vi "TLB Native Dynamic Events ver 0.05g.vi"() -> ()   [LabVIEW 2018]
uses:
  Labview Training Phase 2/Enum Controls/States for Action Engine.ctl
  Type def/TLB event states.ctl
  Type def/TLB MHL States.ctl
  <vilib>/Studica/Studica Toolkit/Background/I2C Channel.ctl
  <vilib>/Studica/Studica Toolkit/NavX/NavX.lvlib
  <vilib>/myRIO/Common/Instrument Driver Framework/myRIO v1.0/AI/typedefs/AI Channels Enum.ctl
  <vilib>/myRIO/Common/Instrument Driver Framework/myRIO v1.0/AI/typedefs/AI Channels List.ctl
  <vilib>/Studica/Studica Toolkit/Background/Mxp Selection.ctl
  <vilib>/ptbypt/NI_PtbyPt.lvlib
  Type def/Type def.ctl
  Type def/Motor Control Cluster.ctl
  <vilib>/Studica/Studica Blackhawk/Blackhawk.lvlib
  <vilib>/vision/driver/NI_Vision_Acquisition_Software.lvlib
  <vilib>/userdefined/High Color/IMAQdx.ctl
panel:
  in  "Enum":T1(ring)
  out "Image Processing error":errorcluster
  out "Image Out":T2(plugin-control)
  out "element":T3
  in  "Servo Angle":u8(slide) scale=0.0..180.0
  in  "On/Off":bool
  out "Blackhawk error":errorcluster
  out "Value Read":bool
  out "Object detected":bool
  out "Yaw":dbl
  in  "NavX Zero Yaw":bool
  out "NavX Info Out":T5
  out "LinearAcceleration":T6
  out "Displacement":T7
  out "YRPHfH":T8
  out "Distance":T9
  in  "Return to IDLE":bool
  out "Right IR Sensor":dbl
  out "Left IR Sensor":dbl
  out "CM":fxp<+,64,16>
  out "Ultrasonic sensor":dbl format="%0.2f"
  in  "xTargetSpeed":dbl
  in  "yTargetSpeed":dbl
  in  "wTargetSpeed":dbl
  out "Speed":T10
  in  "Reset Encoder 0":bool
  out "Action Queue Items":i32
  out "State Logic Queue Items":i32
  out "Action Queues items":string[](array[string])=["Hardware reset", "Software reset", ""]
  out "State logic":T11=enum."Task 2"
  out "Action State":string
  in  "Tasks Selector":string(combo)="Task 2"
  in  "Stop Queue":bool
  in  "Start Task":bool
  # "Test Programme written by Calvin Loke    Dated: 28 Aug 2019\nTest Programme revised by Dr Alex See   Dated 30 Aug 2019\n\nProgramme version:   TLB Native Dynamic Events ver 0.04b.vi"
  # "Sequence of Actions"
  # "Continuous (Repeated)"
  # "System Health Status Update"
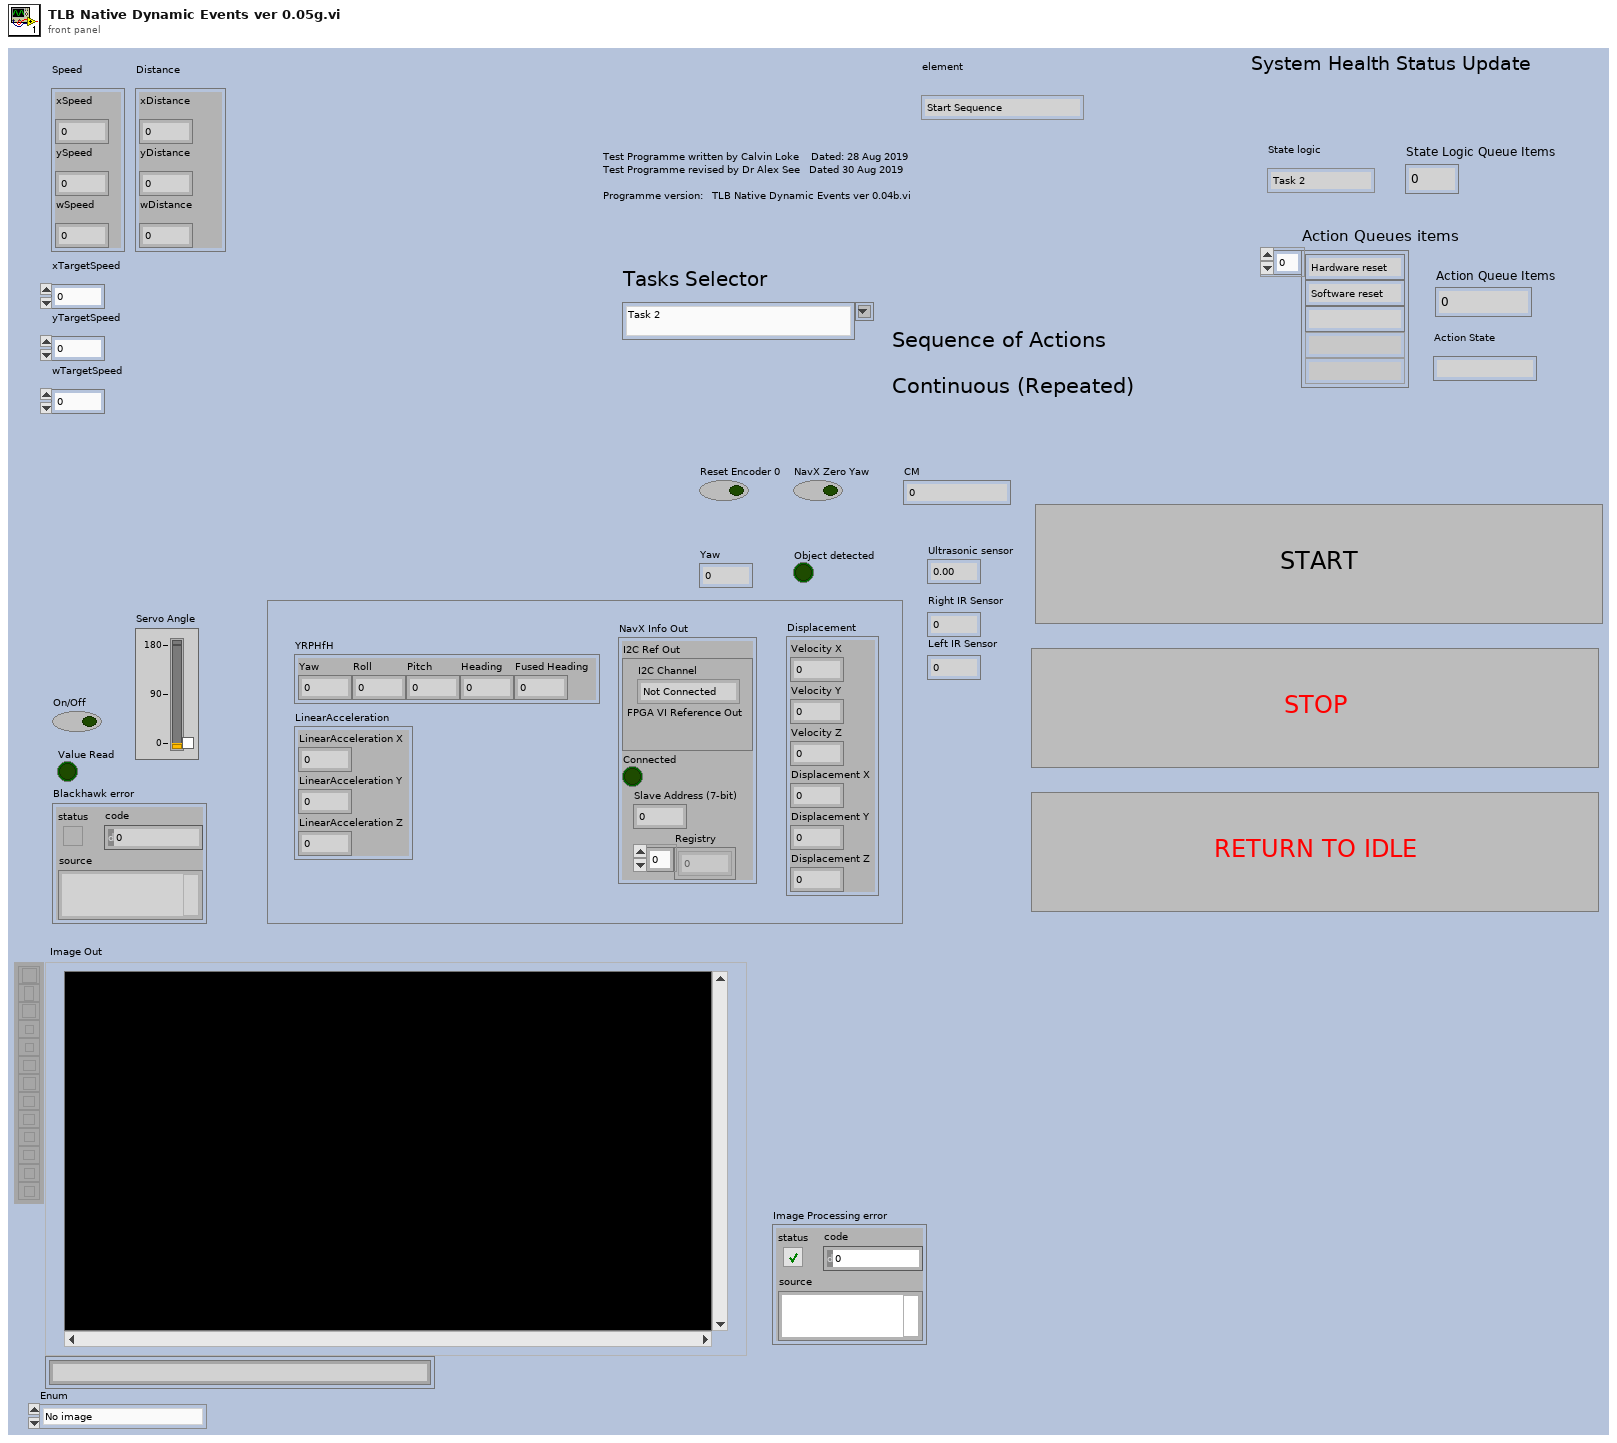
[diagram p1: front panel]
types:
  T1 = enum16{"No image", "Hair gel detection", "Pipe detection", "Ball detection", "Soap detection"}
  T2 = typedef "IMAQ Image.ctl" = refnum<image>
  T3 = typedef "TLB event states.ctl" = enum16{"Start Sequence", "Exit", "Start Task 1", "Start Task 2", "Start Task 3", "Start Task 4", "Camera vision", "Wall follow mode", "Idle", "Start Drive Straight"}
  T4 = typedef "I2C Channel.ctl" = enum16{"Not Connected", "A", "B"}
  T5 = cluster{"I2C Ref Out":cluster{"I2C Channel":T4, "FPGA VI Reference Out":refnum<k20>}, "Connected":bool, "Slave Address (7-bit)":u8, "Registry":u8[]}
  T6 = cluster{"LinearAcceleration X":dbl, "LinearAcceleration Y":dbl, "LinearAcceleration Z":dbl}
  T7 = cluster{"Velocity X":dbl, "Velocity Y":dbl, "Velocity Z":dbl, "Displacement X":dbl, "Displacement Y":dbl, "Displacement Z":dbl}
  T8 = cluster{"Yaw":dbl, "Roll":dbl, "Pitch":dbl, "Heading":dbl, "Fused Heading":dbl}
  T9 = cluster{"xDistance":dbl, "yDistance":dbl, "wDistance":dbl}
  T10 = cluster{"xSpeed":dbl, "ySpeed":dbl, "wSpeed":dbl}
  T11 = typedef "TLB MHL States.ctl" = enum16{"None", "Startup", "Idle", "Processing", "Shutdown", "Reset", "Task 1", "Task 2", "Task 3", "Task 4", "Task 4a", "Task 4b", "Task 4c", "Task 4d", "Task 4e", "Task 4f", "Task 4g", "Task 4h", "Acquire image", "Wall follow mode", "Autodrive", "Autodrive a"}
  T12 = typedef "States for Action Engine.ctl" = enum16{"Initialize", "Write", "Read"}
  T13 = typedef "IMAQdx.ctl" = refnum<k21>
  T14 = typedef "Motor Control Cluster.ctl" = cluster{"Vx":dbl, "Vy":dbl, "Vw":dbl}
  T15 = typedef "Type def.ctl" = cluster{"Front Ultrasonic Obstruct":bool, "Left Ultrasonic Obstruct":bool, "Right Ultrasonic Obstruct ":bool}
  T16 = typedef "Mxp Selection.ctl" = enum16{"MXP A", "MXP B"}
  T17 = typedef "TLB event states.ctl" = enum16{"Start Sequence", "Exit", "Start Task 1", "Start Task 2", "Start Task 3", "Start Task 4", "RT Camera tracking", "Wall follow mode", "Idle"}
  T18 = cluster{"I2C Channel":T4, "FPGA VI Reference Out":refnum<k20>}
  T19 = typedef "AI Channels List.ctl" = T20[]
  T20 = typedef "AI Channels Enum.ctl" = enum16{"Not Connected", "AudioIn/Left", "AudioIn/Right", "C/AI0", "C/AI1", "A/AI0", "A/AI1", "A/AI2", "A/AI3", "A/AI4", "A/AI5", "A/AI6", "A/AI7", "B/AI0", "B/AI1", "B/AI2", "B/AI3", "B/AI4", "B/AI5", "B/AI6", "B/AI7", "AI/AI0", "AI/AI1", "AI/AI2", "AI/AI3", "A/AI0 (DIFF)", "A/AI1 (DIFF)", "A/AI2 (DIFF)", "A/AI3 (DIFF)", "B/AI0 (DIFF)", "B/AI1 (DIFF)", "B/AI2 (DIFF)", "B/AI3 (DIFF)"}
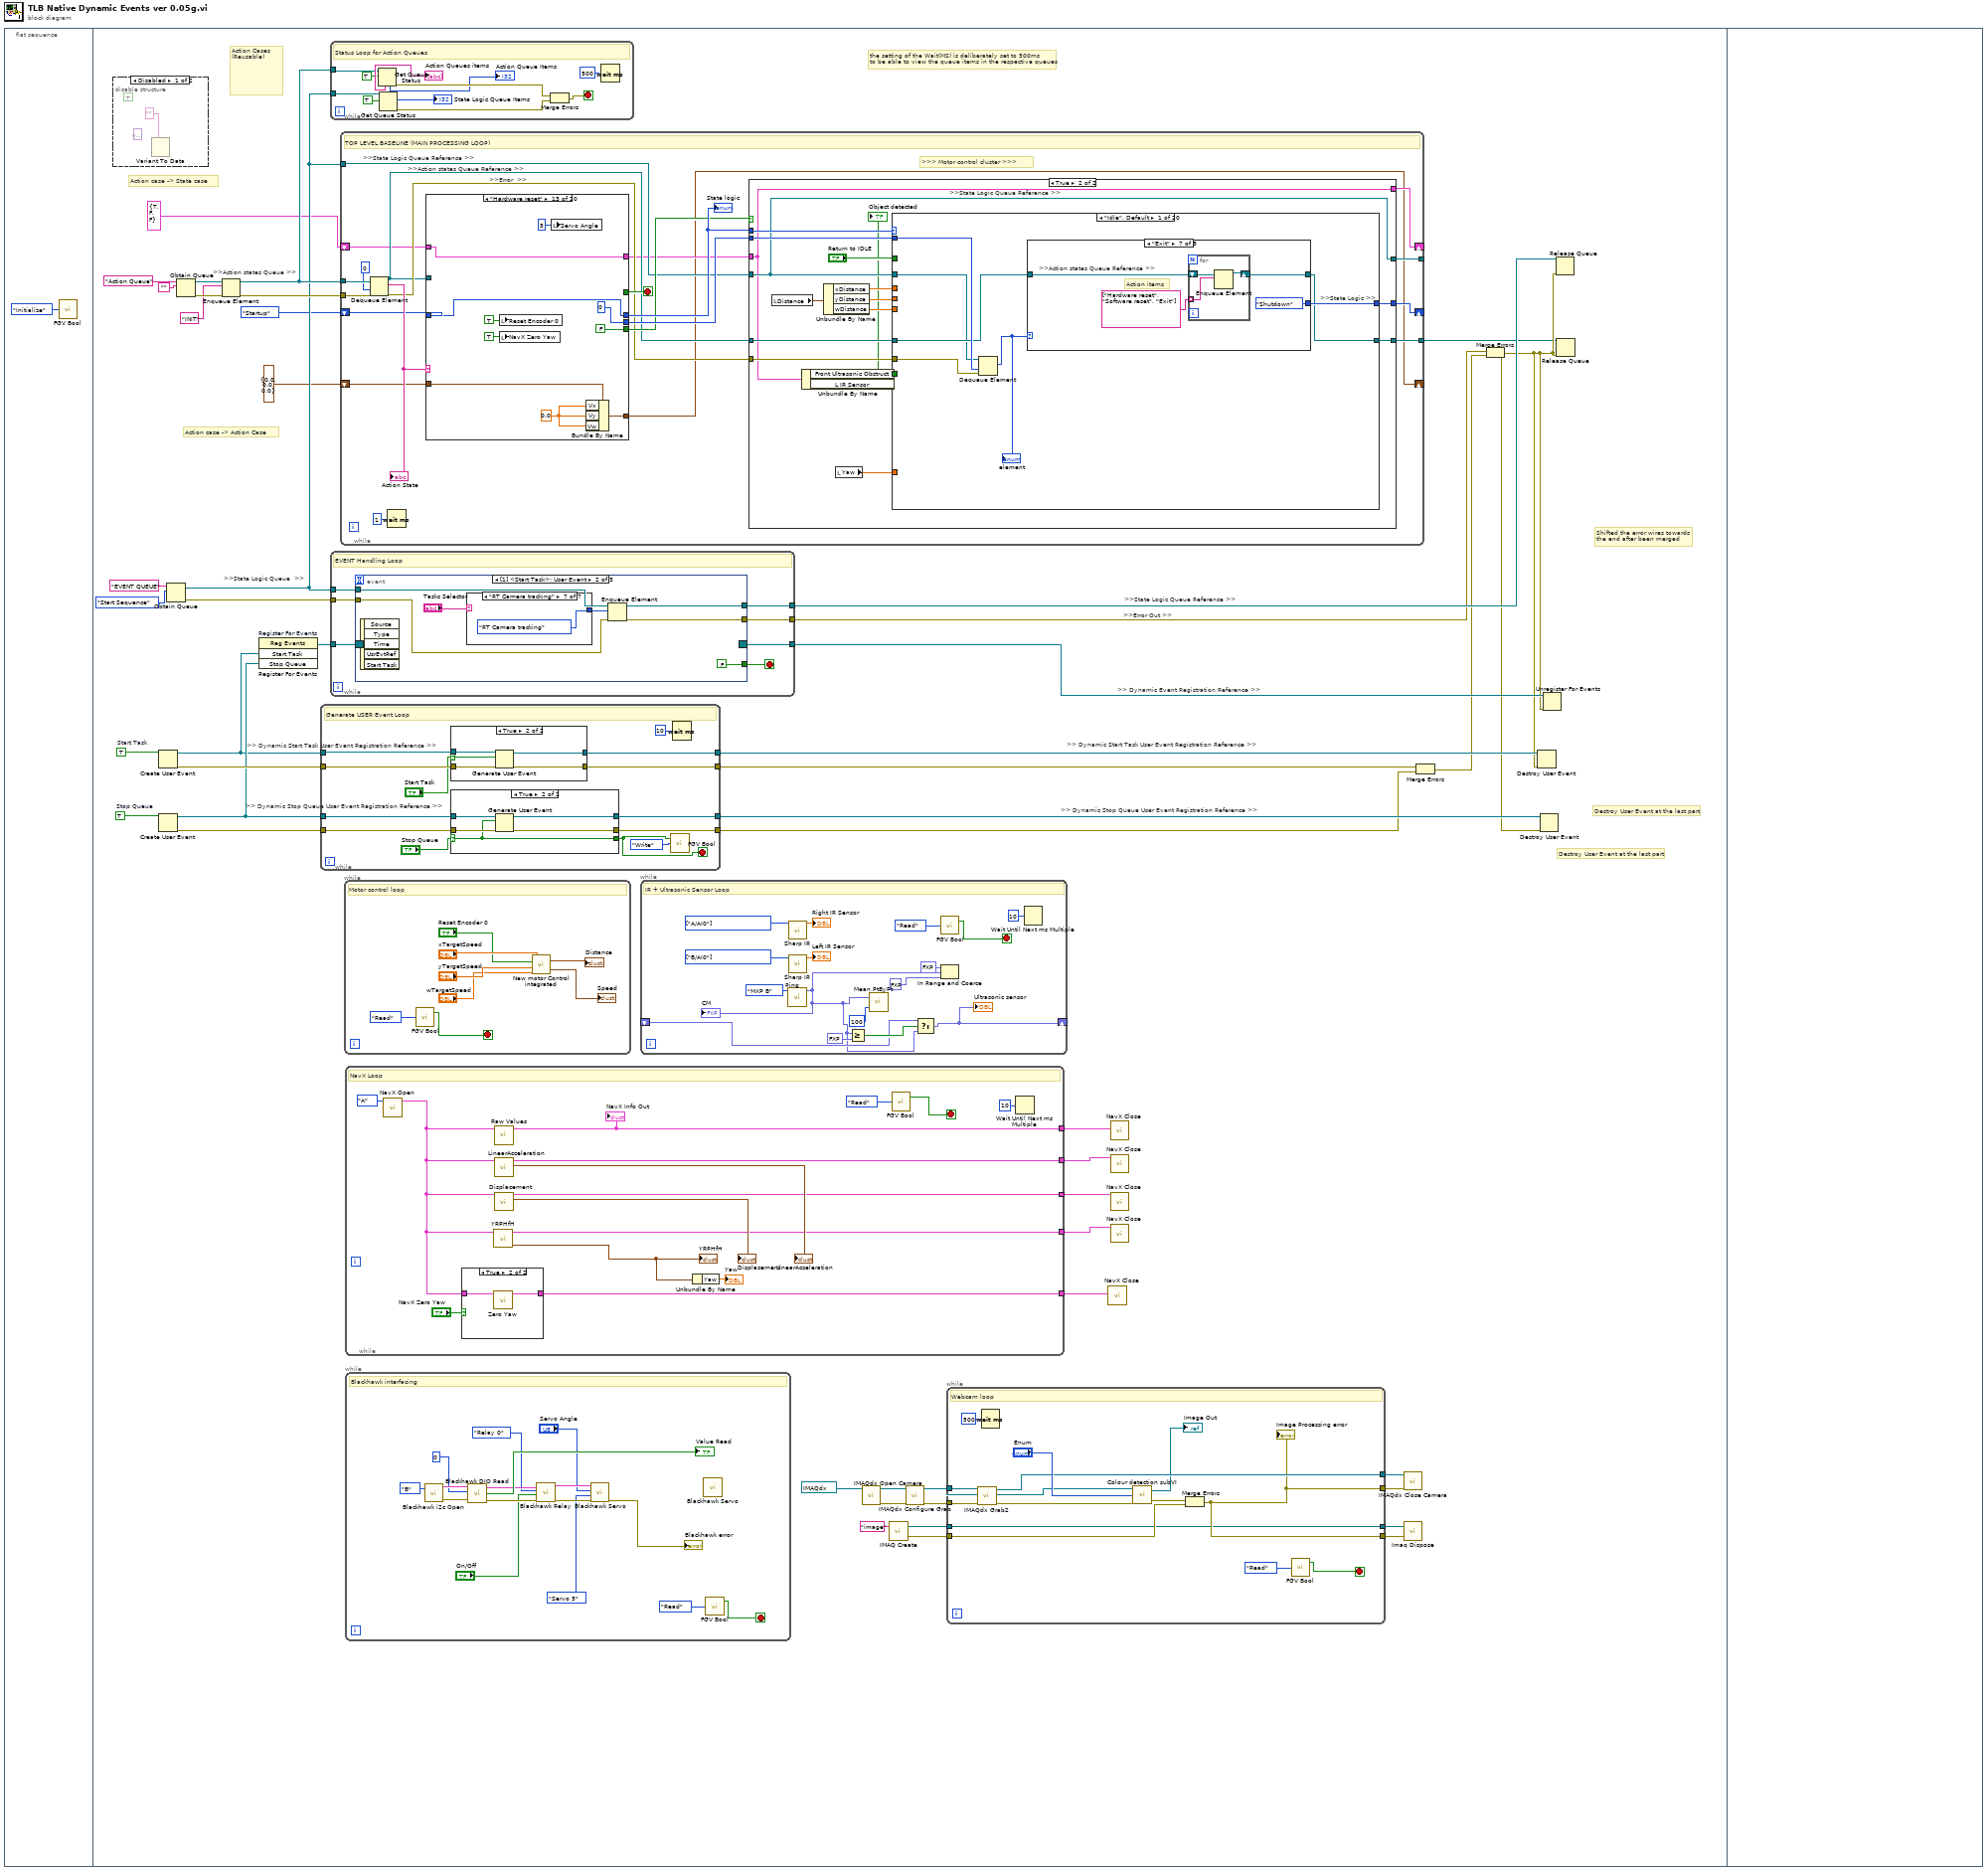
[diagram p0: block diagram]
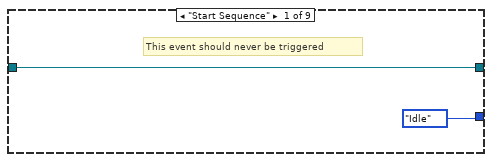
[diagram p5: hidden frame]
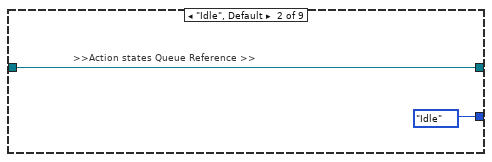
[diagram p6: hidden frame]
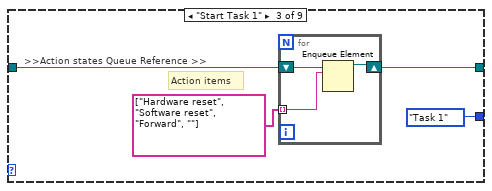
[diagram p7: hidden frame]
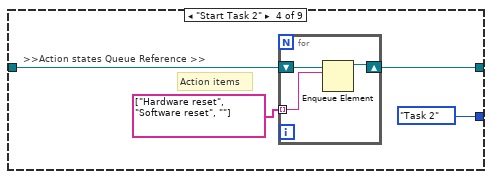
[diagram p8: hidden frame]
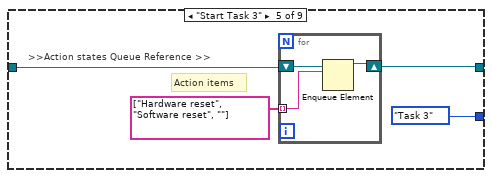
[diagram p9: hidden frame]
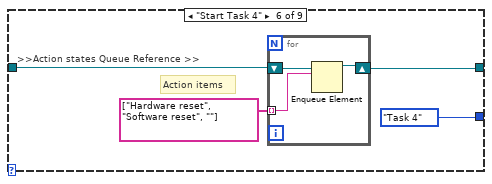
[diagram p10: hidden frame]
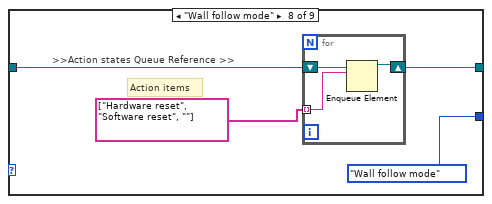
[diagram p11: hidden frame]
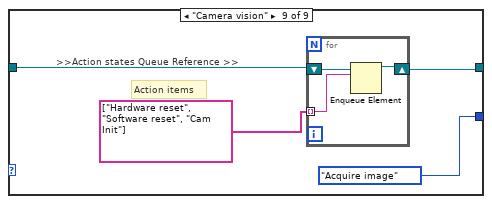
[diagram p12: hidden frame]
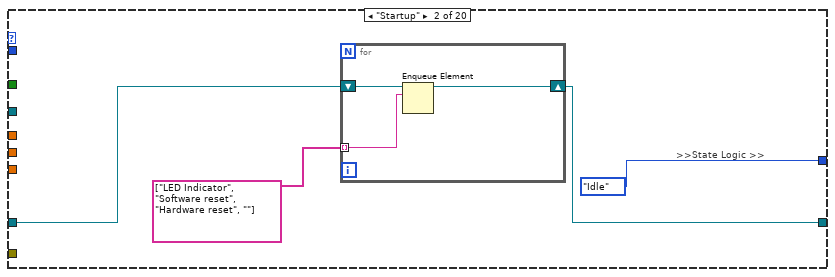
[diagram p13: hidden frame]
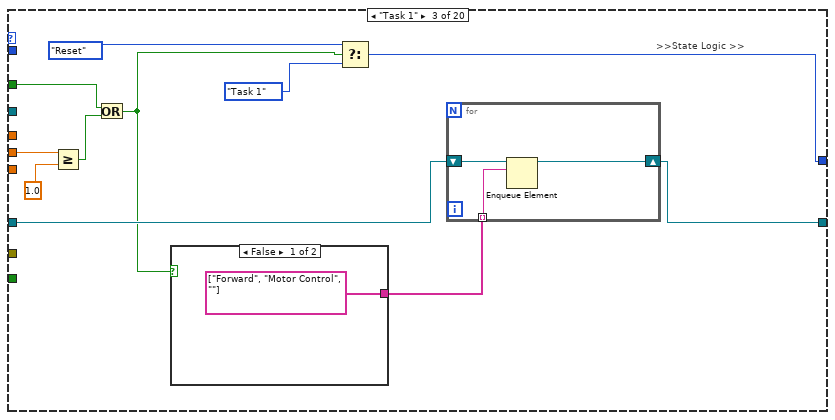
[diagram p14: hidden frame]
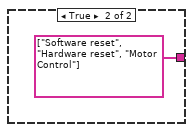
[diagram p15: hidden frame]
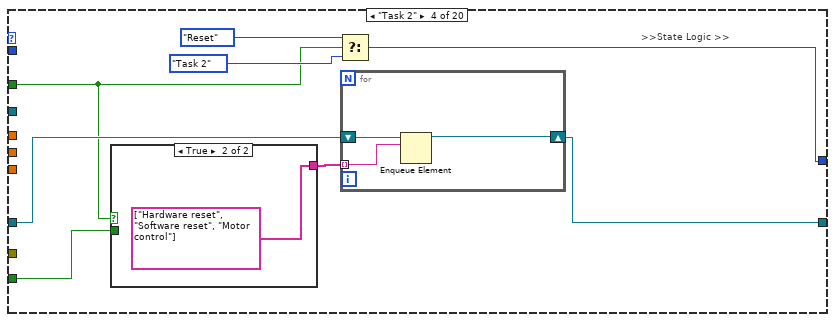
[diagram p16: hidden frame]
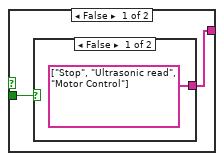
[diagram p17: hidden frame]
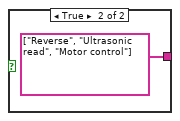
[diagram p18: hidden frame]
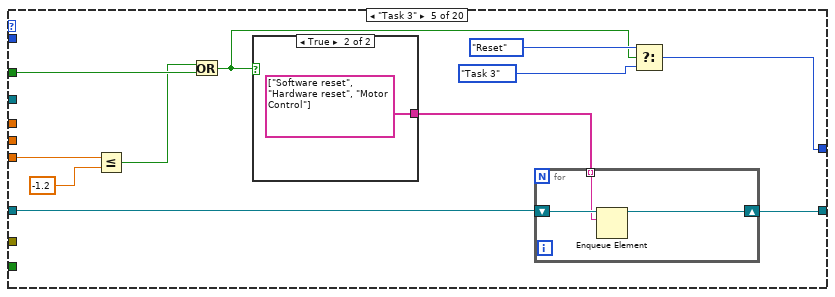
[diagram p19: hidden frame]
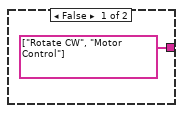
[diagram p20: hidden frame]
diagram:
  n1 = flat-sequence {
    frame #0 {
      n2 = call "FGV Bool.vi"("Init/Read/Write State"=States_for_Action_Engine."Initialize") -> ()  [unwired: 2 in, 2 out]
    }
    frame #1 {
      w49 = TRUE  # Stop Queue
      w48 = TRUE  # Start Task
      # "Action case -> Action Case"
      # "Action case -> State case"
      # "the setting of the Wait(MS) is deliberately set to 500ms\nto be able to view the queue items in the respective queues"
      # "Action Cases\n(Reusable)"
      # ">>Error Out >>"
      # ">> Dynamic Stop Queue User Event Registration Reference >>"
      # ">> Dynamic Start Task User Event Registration Reference >>"
      # ">> Dynamic Stop Queue User Event Registration Reference >>"
      # ">> Dynamic Start Task User Event Registration Reference >>"
      # ">> Dynamic Event Registration Reference >>"
      # ">>Action states Queue >>"
      # ">>State Logic Queue  >>"
      # ">>State Logic Queue Reference >>"
      # "Destroy User Event at the last part"
      # "Destroy User Event at the last part"
      # "Shifted the error wires towards\nthe end after been merged"
      n3 = disable-structure shown="Disabled" {
        frame Disabled {
          (unwired) variant
          (unwired) TRUE
          n4 = Variant To Data(type="") -> ()  [unwired: 2 in, 2 out]
        }
        frame Enabled {
        }
      }
      n5 = Create User Event(user event datatype=w48) -> (user event=w40:refnum<user-event>, error out=w45:errorcluster)  [unwired: 1 in]
      n6 = Create User Event(user event datatype=w49) -> (user event=w41:refnum<user-event>, error out=w44:errorcluster)  [unwired: 1 in]
      n7 = Obtain Queue(name (unnamed)="EVENT QUEUE", element data type=TLB_event_states."Start Sequence" ("Enum")) -> (queue out=w25:refnum<queue>, error out=w31:errorcluster)  [unwired: 3 in, 1 out]
      n8 = Obtain Queue(name (unnamed)="Action Queue", element data type="") -> (queue out=w34:refnum<queue>, error out=w30:errorcluster)  [unwired: 3 in, 1 out]
      n9 = Enqueue Element(queue=w34, element="INIT", error in (no error)=w30) -> (queue out=w26:refnum<queue>, error out=w29:errorcluster)  [unwired: 1 in, 1 out]
      n10 = register-events "Register For Events"(w40, w41) -> (reference out=w39:refnum<event-registration>)  [unwired: 2 in, 1 out]
      n11 = while {
        tunnel: w40 -> [w607]
        tunnel: w41 -> [w606]
        tunnel: [w605] -> w47
        tunnel: [w604] -> w46
        tunnel: w45 -> [w603]
        tunnel: [w602] -> w43
        tunnel: w44 -> [w601]
        tunnel: [w600] -> w42
        stop <- w596 stop-if-true
        # "Generate USER Event Loop"
        n12 = case shown="True" "Start Task" {
          selector: "Start Task" -> [_ w619]
          tunnel: w607 -> [w618 w623]
          tunnel: [w618 w622] -> w604
          tunnel: w603 -> [w617 w621]
          tunnel: [w617 w620] -> w602
          frame False {
          }
          frame True {
            n13 = Generate User Event(user event=w623, event data cluster=w619, error in=w621) -> (user event out=w622:refnum<user-event>, error out=w620:errorcluster)  [unwired: 1 in]
          }
        }
        n14 = case shown="True" "Stop Queue" {
          selector: "Stop Queue" -> [_ w612]
          tunnel: w606 -> [w611 w616]
          tunnel: [w611 w615] -> w605
          tunnel: w601 -> [w610 w614]
          tunnel: [w610 w613] -> w600
          tunnel: [FALSE w612] -> w596
          frame False {
          }
          frame True {
            n15 = Generate User Event(user event=w616, event data cluster=w612, error in=w614) -> (user event out=w615:refnum<user-event>, error out=w613:errorcluster)  [unwired: 1 in]
          }
        }
        n16 = call "FGV Bool.vi"("Init/Read/Write State"=States_for_Action_Engine."Write", "Input Node"=w596) -> ()  [unwired: 1 in, 2 out]
        n17 = Wait (ms)(milliseconds to wait=u32 10) -> ()  [unwired: 1 out]
      }
      n18 = while {
        tunnel: w26 -> [w131]
        tunnel: w25 -> [w128]
        stop <- w125 stop-if-true
        # "Status Loop for Action Queues"
        n19 = Get Queue Status(queue=w131, return elements? (F)=TRUE) -> (error out=w127:errorcluster, # elements in queue=→"Action Queue Items":i32, elements=→"Action Queues items":string[])  [unwired: 1 in, 5 out]
        n20 = Get Queue Status(queue=w128, return elements? (F)=TRUE) -> (# pending remove=→"State Logic Queue Items":i32, error out=w126:errorcluster)  [unwired: 1 in, 6 out]
        n21 = Merge Errors(w127, w126) -> (w125:errorcluster)
        n22 = Wait (ms)(milliseconds to wait=u32 500) -> ()  [unwired: 1 out]
      }
      n23 = while {
        tunnel: w39 -> [w569]
        tunnel: [w568] -> w38
        tunnel: w25 -> [w566]
        tunnel: [w565] -> w37
        tunnel: w31 -> [w564]
        tunnel: [w563] -> w28
        stop <- w567 stop-if-true
        # "EVENT Handling Loop"
        n24 = event shown="[1] <Start Task>: User Event" {
          selector: w569 -> [_ _ _]
          dyn-events: [_ _ _] -> w568
          timeout: _ -> [_ _ _]
          tunnel: [FALSE FALSE w595] -> w567
          tunnel: w566 -> [w574 w581 w593]
          tunnel: [w573 w580 w594] -> w565
          tunnel: w564 -> [w571 w577 w591]
          tunnel: [w570 w576 w590] -> w563
          event Timeout {
            n25 = event-data() -> ()  [unwired: 1 in, 3 out]
            n26 = Enqueue Element(queue=w574, element=TLB_event_states."Idle" ("Enum"), error in (no error)=w571) -> (queue out=w573:refnum<queue>, error out=w570:errorcluster)  [unwired: 1 in, 1 out]
          }
          event User Event {
            n27 = event-data() -> ()  [unwired: 1 in, 5 out]
            n28 = case shown="\"RT Camera tracking\"" "Tasks Selector" {
              tunnel: [TLB_event_states."Idle" ("Enum") TLB_event_states."Start Task 1" ("Enum") TLB_event_states."Start Task 2" ("Enum") TLB_event_states."Start Task 3" ("Enum") TLB_event_states."Start Task 4" ("Enum") TLB_event_states."Wall follow mode" ("Enum") TLB_event_states."RT Camera tracking" ("Enum")] -> w578
              frame Default {
              }
              frame "Task 1" {
              }
              frame "Task 2" {
              }
              frame "Task 3" {
              }
              frame "Task 4" {
              }
              frame "Wall following" {
              }
              frame "RT Camera tracking" {
              }
            }
            n29 = Enqueue Element(queue=w581, element=w578, error in (no error)=w577) -> (queue out=w580:refnum<queue>, error out=w576:errorcluster)  [unwired: 1 in, 1 out]
          }
          event User Event {
            n30 = event-data() -> ("Stop Queue"=w595:bool)  [unwired: 1 in, 4 out]
            n31 = Enqueue Element At Opposite End(queue=w593, element=TLB_event_states."Exit" ("Enum"), error in (no error)=w591) -> (queue out=w594:refnum<queue>, error out=w590:errorcluster)  [unwired: 1 in, 1 out]
          }
        }
      }
      n32 = while {
        tunnel: w25 -> [w142]
        shift-right: [w147] -> _
        shift-left: TLB_MHL_States."Startup" ("Enum") -> [w139]
        tunnel: w26 -> [w152]
        tunnel: w29 -> [w150]
        tunnel: [w149] -> _
        tunnel: [w148] -> w23
        shift-right: [w136] -> _
        shift-left: T15 {"Front Ultrasonic Obstruct"=TRUE, "Left Ultrasonic Obstruct"=FALSE, "Right Ultrasonic Obstruct "=FALSE} -> [w138]
        shift-right: [w134] -> _
        shift-left: T14 {"Vx"=0.0, "Vy"=0.0, "Vw"=0.0} -> [w135]
        stop <- w145 stop-if-true
        # ">>> Motor control cluster >>>"
        # ">>Error  >>"
        # ">>Action states Queue Reference >>"
        # ">>State Logic Queue Reference >>"
        # "TOP LEVEL BASELINE (MAIN PROCESSING LOOP)"
        n33 = Dequeue Element(queue=w152, timeout in ms (-1)=0, error in (no error)=w150) -> (queue out=w140:refnum<queue>, element=w151:string, error out=w141:errorcluster)  [unwired: 1 out]
        "Action State" <- w151
        n34 = Wait (ms)(milliseconds to wait=u32 1) -> ()  [unwired: 1 out]
        n35 = case shown="\"Hardware reset\"" w151 {
          tunnel: [w409 w417 w422 w430 w439 w449 w458 w465 w476 w484 w492 w501 w511 TLB_MHL_States."Shutdown" ("Enum") w526 w530 w544 w550 w553 w562] -> w153
          tunnel: [w408 0 0 0 0 0 0 0 0 0 0 0 0 0 0 0 0 0 0 0] -> w146
          tunnel: [_ _ _ _ _ _ _ _ _ _ _ _ _ TRUE _ _ _ _ _ _] -> w145
          tunnel: [TRUE FALSE FALSE FALSE FALSE FALSE FALSE FALSE FALSE FALSE FALSE FALSE FALSE FALSE FALSE FALSE FALSE FALSE FALSE FALSE] -> w144
          tunnel: w140 -> [_ _ _ _ _ _ _ _ _ _ _ _ _ _ _ _ _ _ _ _]
          tunnel: w139 -> [w409 w417 w422 w430 w439 w449 w458 w465 w476 w484 w492 w501 w511 _ w526 w530 w544 w550 w553 w562]
          tunnel: w138 -> [w406 w414 w419 w426 w435 w444 w453 w462 w471 w480 w493 w498 w506 w513 w525 w533 w545 w551 w552 w558]
          tunnel: [w406 w414 w419 w426 w435 w444 w453 w462 w471 w480 w493 w497 w506 w513 w522 w532 w545 w551 w552 w558] -> w137
          tunnel: w135 -> [w405 w413 w418 w424 w433 w442 w452 w460 w470 w478 w486 w495 w505 w512 w518 w527 w536 w549 w556 w559]
          tunnel: [w405 w413 w418 w425 w434 w443 w451 w461 w469 w479 w486 w495 w503 w512 w518 w527 w537 w549 w556 w559] -> w134
          frame "No action", Default {
            n36 = case shown="\"Startup\", Default" w409 {
              tunnel: [0 100] -> w408
              frame "Startup", Default {
              }
              frame "Idle" {
              }
            }
          }
          frame "Init" {
            # ">>State Logic  >>"
            n37 = local write "Servo Angle"(u8 112 ("Servo Angle")) -> ()
          }
          frame "LED Indicator" {
          }
          frame "Forward" {
            n38 = local write "Reset Encoder 0"(FALSE ("Reset Encoder 0")) -> ()
            n39 = local write "NavX Zero Yaw"(FALSE ("NavX Zero Yaw")) -> ()
            n40 = Bundle By Name(cluster=w424, "Vy"=0.6) -> (w425:T14)
          }
          frame "Reverse" {
            n41 = local write "NavX Zero Yaw"(FALSE ("NavX Zero Yaw")) -> ()
            n42 = local write "Reset Encoder 0"(FALSE ("Reset Encoder 0")) -> ()
            n43 = Bundle By Name(cluster=w433, "Vy"=-0.6) -> (w434:T14)
          }
          frame "Right" {
            n44 = local write "NavX Zero Yaw"(FALSE ("NavX Zero Yaw")) -> ()
            n45 = local write "Reset Encoder 0"(FALSE ("Reset Encoder 0")) -> ()
            n46 = Bundle By Name(cluster=w442, "Vx"=0.6) -> (w443:T14)
          }
          frame "Left" {
            n47 = Bundle By Name(cluster=w452, "Vx"=-0.6) -> (w451:T14)
            n48 = local write "NavX Zero Yaw"(FALSE ("NavX Zero Yaw")) -> ()
            n49 = local write "Reset Encoder 0"(FALSE ("Reset Encoder 0")) -> ()
          }
          frame "Rotate CW" {
            n50 = local write "NavX Zero Yaw"(FALSE ("NavX Zero Yaw")) -> ()
            n51 = local write "Reset Encoder 0"(FALSE ("Reset Encoder 0")) -> ()
            n52 = Bundle By Name(cluster=w460, "Vw"=-0.3) -> (w461:T14)
          }
          frame "Rotate ACW" {
            n53 = local write "Reset Encoder 0"(FALSE ("Reset Encoder 0")) -> ()
            n54 = local write "NavX Zero Yaw"(FALSE ("NavX Zero Yaw")) -> ()
            n55 = Bundle By Name(cluster=w470, "Vw"=0.15) -> (w469:T14)
          }
          frame "Stop" {
            w477 = 0.0
            n56 = local write "NavX Zero Yaw"(FALSE ("NavX Zero Yaw")) -> ()
            n57 = local write "Reset Encoder 0"(FALSE ("Reset Encoder 0")) -> ()
            n58 = Bundle By Name(cluster=w478, "Vx"=w477, "Vy"=w477, "Vw"=w477) -> (w479:T14)
          }
          frame "Motor control" {
            # "Replace with FGV"
            n59 = Unbundle By Name(w486) -> ("Vx"=w489:dbl, "Vy"=w488:dbl, "Vw"=w487:dbl)
            n60 = local write "xTargetSpeed"(w489) -> ()
            n61 = local write "yTargetSpeed"(w488) -> ()
            n62 = local write "wTargetSpeed"(w487) -> ()
          }
          frame "Software reset" {
            w496 = FALSE ("NavX Zero Yaw")
            n63 = local write "NavX Zero Yaw"(w496) -> ()
            n64 = Bundle By Name(cluster=w498, "Front Ultrasonic Obstruct"=w496, "L IR Sensor"=0.0) -> (w497:T15)
          }
          frame "Hardware reset" {
            w504 = 0.0
            n65 = local write "Reset Encoder 0"(TRUE ("Reset Encoder 0")) -> ()
            n66 = local write "NavX Zero Yaw"(TRUE ("NavX Zero Yaw")) -> ()
            n67 = local write "Servo Angle"(u8 5 ("Servo Angle")) -> ()
            n68 = Bundle By Name(cluster=w505, "Vx"=w504, "Vy"=w504, "Vw"=w504) -> (w503:T14)
          }
          frame "Exit" {
          }
          frame "Ultrasonic read" {
            # "Object detection"
            n69 = local read "Ultrasonic sensor"() -> (w521:dbl)
            n70 = Less Or Equal?(x=w521, y=20.0) -> (x <= y?=w519:bool)
            n71 = Bundle By Name(cluster=w525, "Front Ultrasonic Obstruct"=w519) -> (w522:T15)
          }
          frame "IR Sensor Read" {
            n72 = local read "Left IR Sensor"() -> (w531:dbl)
            n73 = Bundle By Name(cluster=w533, "L IR Sensor"=w531) -> (w532:T15)
          }
          frame "Calculate" {
            n74 = Unbundle By Name(w545) -> ("L IR Sensor"=w541:dbl)
            n75 = Subtract(x=w541, y=20.0) -> (x-y=w539:dbl)
            n76 = Multiply(x=w539, y=0.01) -> (x*y=w535:dbl)
            n77 = Bundle By Name(cluster=w536, "Vy"=0.4, "Vw"=w535) -> (w537:T14)
          }
          frame "Cam Init" {
            n78 = local write "Servo Angle"(u8 5 ("Servo Angle")) -> ()
          }
          frame "Cam Acq" {
          }
          frame "Cam Exit" {
            n79 = local write "Servo Angle"(u8 112 ("Servo Angle")) -> ()
          }
        }
        "State logic" <- w153
        n80 = case shown="True" w144 {
          tunnel: w153 -> [w157 w173]
          tunnel: w142 -> [w158 w167]
          tunnel: w140 -> [w156 w172]
          tunnel: [w158 w167] -> w149
          tunnel: [w156 w171] -> w148
          tunnel: [w157 w170] -> w147
          tunnel: w141 -> [_ w169]
          tunnel: w146 -> [_ w168]
          tunnel: w137 -> [w155 w159]
          tunnel: [w155 w159] -> w136
          frame False {
          }
          frame True {
            # ">>State Logic Queue Reference >>"
            n81 = local read "Distance"() -> (w165:T9)
            n82 = Unbundle By Name(w159) -> ("Front Ultrasonic Obstruct"=w160:bool)  [unwired: 1 out]
            "Object detected" <- w160
            n83 = Unbundle By Name(w165) -> ("xDistance"=w162:dbl, "yDistance"=w164:dbl, "wDistance"=w163:dbl)
            n84 = local read "Yaw"() -> (w161:dbl)
            n85 = case shown="\"Idle\", Default" w173 {
              tunnel: w167 -> [w174 _ _ _ _ _ _ _ _ _ _ _ _ _ _ _ _ _ _ _]
              tunnel: w172 -> [w176 w235 w247 w260 w282 w291 w305 w320 w333 w346 w357 w363 w366 w372 w375 w377 w379 w381 w384 w397]
              tunnel: [w175 w234 w246 w261 w281 w292 w304 w319 w332 w345 w356 w363 w365 w372 w375 w377 w379 w381 w385 w396] -> w171
              tunnel: [w179 TLB_MHL_States."Idle" ("Enum") w249 w262 w278 w295 w307 w318 w334 w344 TLB_MHL_States."Idle" ("Enum") TLB_MHL_States."Reset" ("Enum") TLB_MHL_States."Shutdown" ("Enum") TLB_MHL_States."Reset" ("Enum") TLB_MHL_States."Idle" ("Enum") TLB_MHL_States."Idle" ("Enum") TLB_MHL_States."Idle" ("Enum") TLB_MHL_States."Idle" ("Enum") w387 w395] -> w170
              tunnel: w169 -> [w177 _ _ _ _ _ _ _ _ _ _ _ _ _ _ _ _ _ _ _]
              tunnel: w168 -> [w178 _ _ _ _ _ _ _ _ _ _ _ _ _ _ _ _ _ _ _]
              tunnel: "Return to IDLE" -> [_ _ w244 w259 w276 _ _ _ _ _ _ _ _ _ _ _ _ _ w382 w394]
              tunnel: w164 -> [_ _ w243 _ _ _ _ w317 _ _ _ _ _ _ _ _ _ _ _ _]
              tunnel: w163 -> [_ _ _ _ w275 _ _ _ _ _ _ _ _ _ _ _ _ _ _ _]
              tunnel: w162 -> [_ _ _ _ _ _ w301 _ w329 _ _ _ _ _ _ _ _ _ _ _]
              tunnel: w161 -> [_ _ _ _ _ _ _ _ _ _ _ _ _ _ _ _ _ _ _ _]
              tunnel: w160 -> [_ _ _ w257 _ w289 _ _ _ w343 _ _ _ _ _ _ _ _ _ _]
              frame "Idle", Default {
                # ">>State Logic >>"
                n86 = Dequeue Element(queue=w174, timeout in ms (-1)=w178, error in (no error)=w177) -> (element=w180:T3)  [unwired: 3 out]
                "element" <- w180
                n87 = case shown="\"Exit\"" w180 {
                  tunnel: [TLB_MHL_States."Idle" ("Enum") TLB_MHL_States."Idle" ("Enum") TLB_MHL_States."Task 1" ("Enum") TLB_MHL_States."Task 2" ("Enum") TLB_MHL_States."Task 3" ("Enum") TLB_MHL_States."Task 4" ("Enum") TLB_MHL_States."Shutdown" ("Enum") TLB_MHL_States."Wall follow mode" ("Enum") TLB_MHL_States."Acquire image" ("Enum")] -> w179
                  tunnel: [w182 w183 w187 w192 w201 w207 w213 w220 w228] -> w175
                  tunnel: w176 -> [w182 w183 w185 w193 w202 w208 w214 w221 w229]
                  frame "Start Sequence" {
                    # "This event should never be triggered"
                  }
                  frame "Idle", Default {
                    # ">>Action states Queue Reference >>"
                  }
                  frame "Start Task 1" {
                    # ">>Action states Queue Reference >>"
                    # "Action items"
                    n88 = for {
                      shift-right: [w191] -> w187
                      shift-left: w185 -> [w190]
                      tunnel: string[] ["Hardware reset", "Software reset", "Forward", ""] -> [w189] mode=indexing
                      n89 = Enqueue Element(queue=w190, element=w189) -> (queue out=w191:refnum<queue>)  [unwired: 2 in, 2 out]
                    }
                  }
                  frame "Start Task 2" {
                    # ">>Action states Queue Reference >>"
                    # "Action items"
                    n90 = for {
                      shift-right: [w198] -> w192
                      shift-left: w193 -> [w197]
                      tunnel: string[] ["Hardware reset", "Software reset", ""] -> [w196] mode=indexing
                      n91 = Enqueue Element(queue=w197, element=w196) -> (queue out=w198:refnum<queue>)  [unwired: 2 in, 2 out]
                    }
                  }
                  frame "Start Task 3" {
                    # ">>Action states Queue Reference >>"
                    # "Action items"
                    n92 = for {
                      shift-right: [w205] -> w201
                      shift-left: w202 -> [w204]
                      tunnel: string[] ["Hardware reset", "Software reset", ""] -> [w203] mode=indexing
                      n93 = Enqueue Element(queue=w204, element=w203) -> (queue out=w205:refnum<queue>)  [unwired: 2 in, 2 out]
                    }
                  }
                  frame "Start Task 4" {
                    # ">>Action states Queue Reference >>"
                    # "Action items"
                    n94 = for {
                      shift-right: [w212] -> w207
                      shift-left: w208 -> [w211]
                      tunnel: string[] ["Hardware reset", "Software reset", ""] -> [w210] mode=indexing
                      n95 = Enqueue Element(queue=w211, element=w210) -> (queue out=w212:refnum<queue>)  [unwired: 2 in, 2 out]
                    }
                  }
                  frame "Exit" {
                    # ">>Action states Queue Reference >>"
                    # "Action items"
                    n96 = for {
                      shift-right: [w219] -> w213
                      shift-left: w214 -> [w218]
                      tunnel: string[] ["Hardware reset", "Software reset", "Exit"] -> [w217] mode=indexing
                      n97 = Enqueue Element(queue=w218, element=w217) -> (queue out=w219:refnum<queue>)  [unwired: 2 in, 2 out]
                    }
                  }
                  frame "Wall follow mode" {
                    # ">>Action states Queue Reference >>"
                    # "Action items"
                    n98 = for {
                      shift-right: [w226] -> w220
                      shift-left: w221 -> [w225]
                      tunnel: string[] ["Hardware reset", "Software reset", ""] -> [w224] mode=indexing
                      n99 = Enqueue Element(queue=w225, element=w224) -> (queue out=w226:refnum<queue>)  [unwired: 2 in, 2 out]
                    }
                  }
                  frame "Camera vision" {
                    # ">>Action states Queue Reference >>"
                    # "Action items"
                    n100 = for {
                      shift-right: [w233] -> w228
                      shift-left: w229 -> [w232]
                      tunnel: string[] ["Hardware reset", "Software reset", "Cam Init"] -> [w231] mode=indexing
                      n101 = Enqueue Element(queue=w232, element=w231) -> (queue out=w233:refnum<queue>)  [unwired: 2 in, 2 out]
                    }
                  }
                }
              }
              frame "Startup" {
                # ">>State Logic >>"
                n102 = for {
                  shift-right: [w239] -> w234
                  shift-left: w235 -> [w240]
                  tunnel: string[] ["LED Indicator", "Software reset", "Hardware reset", ""] -> [w238] mode=indexing
                  n103 = Enqueue Element(queue=w240, element=w238) -> (queue out=w239:refnum<queue>)  [unwired: 2 in, 2 out]
                }
              }
              frame "Task 1" {
                # ">>State Logic >>"
                n104 = Greater Or Equal?(x=w243, y=1.0) -> (x >= y?=w241:bool)
                n105 = Or(x=w244, y=w241) -> (x .or. y?=w245:bool)
                n106 = case shown="False" w245 {
                  tunnel: [string[] ["Forward", "Motor Control", ""] string[] ["Software reset", "Hardware reset", "Motor Control"]] -> w248
                  frame False {
                  }
                  frame True {
                  }
                }
                n107 = Select(t=TLB_MHL_States."Reset" ("Enum"), s=w245, f=TLB_MHL_States."Task 1" ("Enum")) -> (s? t:f=w249:T11)
                n108 = for {
                  shift-right: [w255] -> w246
                  shift-left: w247 -> [w256]
                  tunnel: w248 -> [w254] mode=indexing
                  n109 = Enqueue Element(queue=w256, element=w254) -> (queue out=w255:refnum<queue>)  [unwired: 2 in, 2 out]
                }
              }
              frame "Task 2" {
                # ">>State Logic >>"
                n110 = case shown="True" w259 {
                  tunnel: [w266 string[] ["Hardware reset", "Software reset", "Motor control"]] -> w258
                  tunnel: w257 -> [w265 _]
                  frame False {
                    n111 = case shown="False" w265 {
                      tunnel: [string[] ["Stop", "Ultrasonic read", "Motor Control"] string[] ["Reverse", "Ultrasonic read", "Motor control"]] -> w266
                      frame False {
                      }
                      frame True {
                      }
                    }
                  }
                  frame True {
                  }
                }
                n112 = Select(t=TLB_MHL_States."Reset" ("Enum"), s=w259, f=TLB_MHL_States."Task 2" ("Enum")) -> (s? t:f=w262:T11)
                n113 = for {
                  shift-right: [w271] -> w261
                  shift-left: w260 -> [w272]
                  tunnel: w258 -> [w270] mode=indexing
                  n114 = Enqueue Element(queue=w272, element=w270) -> (queue out=w271:refnum<queue>)  [unwired: 2 in, 2 out]
                }
              }
              frame "Task 3" {
                n115 = Less Or Equal?(x=w275, y=-1.2) -> (x <= y?=w273:bool)
                n116 = Or(x=w273, y=w276) -> (x .or. y?=w277:bool)
                n117 = case shown="True" w277 {
                  tunnel: [string[] ["Rotate CW", "Motor Control"] string[] ["Software reset", "Hardware reset", "Motor Control"]] -> w283
                  frame False {
                  }
                  frame True {
                  }
                }
                n118 = for {
                  shift-right: [w285] -> w281
                  shift-left: w282 -> [w286]
                  tunnel: w283 -> [w284] mode=indexing
                  n119 = Enqueue Element(queue=w286, element=w284) -> (queue out=w285:refnum<queue>)  [unwired: 2 in, 2 out]
                }
                n120 = Select(t=TLB_MHL_States."Reset" ("Enum"), s=w277, f=TLB_MHL_States."Task 3" ("Enum")) -> (s? t:f=w278:T11)
              }
              frame "Task 4" {
                n121 = case shown="False" w289 {
                  tunnel: [string[] ["Forward", "Ultrasonic read", "Motor Control"] string[] ["Stop", "Hardware reset", "Software reset", "Motor Control"]] -> w290
                  frame False {
                  }
                  frame True {
                  }
                }
                n122 = for {
                  shift-right: [w299] -> w292
                  shift-left: w291 -> [w300]
                  tunnel: w290 -> [w298] mode=indexing
                  n123 = Enqueue Element(queue=w300, element=w298) -> (queue out=w299:refnum<queue>)  [unwired: 2 in, 2 out]
                }
                n124 = Select(t=TLB_MHL_States."Task 4a" ("Enum"), s=w289, f=TLB_MHL_States."Task 4" ("Enum")) -> (s? t:f=w295:T11)
              }
              frame "Task 4a" {
                n125 = Greater Or Equal?(x=w301, y=0.5) -> (x >= y?=w303:bool)
                n126 = case shown="True" w303 {
                  tunnel: [string[] ["Right", "Motor Control"] string[] ["Stop", "Hardware reset", "Software reset", "Motor Control"]] -> w306
                  frame False {
                  }
                  frame True {
                  }
                }
                n127 = for {
                  shift-right: [w313] -> w304
                  shift-left: w305 -> [w314]
                  tunnel: w306 -> [w312] mode=indexing
                  n128 = Enqueue Element(queue=w314, element=w312) -> (queue out=w313:refnum<queue>)  [unwired: 2 in, 2 out]
                }
                n129 = Select(t=TLB_MHL_States."Task 4b" ("Enum"), s=w303, f=TLB_MHL_States."Task 4a" ("Enum")) -> (s? t:f=w307:T11)
              }
              frame "Task 4b" {
                n130 = Greater Or Equal?(x=w317, y=0.75) -> (x >= y?=w315:bool)
                n131 = case shown="False" w315 {
                  tunnel: [string[] ["Forward", "Motor control"] string[] ["Stop", "Hardware reset", "Software reset"]] -> w321
                  frame False {
                  }
                  frame True {
                  }
                }
                n132 = for {
                  shift-right: [w327] -> w319
                  shift-left: w320 -> [w328]
                  tunnel: w321 -> [w326] mode=indexing
                  n133 = Enqueue Element(queue=w328, element=w326) -> (queue out=w327:refnum<queue>)  [unwired: 2 in, 2 out]
                }
                n134 = Select(t=TLB_MHL_States."Task 4c" ("Enum"), s=w315, f=TLB_MHL_States."Task 4b" ("Enum")) -> (s? t:f=w318:T11)
              }
              frame "Task 4c" {
                n135 = Less Or Equal?(x=w329, y=-0.65) -> (x <= y?=w330:bool)
                n136 = case shown="False" w330 {
                  tunnel: [string[] ["Left"] string[] ["Stop", "Hardware reset", "Software reset"]] -> w335
                  frame False {
                  }
                  frame True {
                  }
                }
                n137 = for {
                  shift-right: [w341] -> w332
                  shift-left: w333 -> [w342]
                  tunnel: w335 -> [w340] mode=indexing
                  n138 = Enqueue Element(queue=w342, element=w340) -> (queue out=w341:refnum<queue>)  [unwired: 2 in, 2 out]
                }
                n139 = Select(t=TLB_MHL_States."Task 4d" ("Enum"), s=w330, f=TLB_MHL_States."Task 4c" ("Enum")) -> (s? t:f=w334:T11)
              }
              frame "Task 4d" {
                n140 = case shown="False" w343 {
                  tunnel: [string[] ["Forward", "Ultrasonic Read"] string[] ["Stop", "Hardware reset", "Software reset"]] -> w347
                  frame False {
                  }
                  frame True {
                  }
                }
                n141 = for {
                  shift-right: [w353] -> w345
                  shift-left: w346 -> [w354]
                  tunnel: w347 -> [w352] mode=indexing
                  n142 = Enqueue Element(queue=w354, element=w352) -> (queue out=w353:refnum<queue>)  [unwired: 2 in, 2 out]
                }
                n143 = Select(t=TLB_MHL_States."Task 4e" ("Enum"), s=w343, f=TLB_MHL_States."Task 4d" ("Enum")) -> (s? t:f=w344:T11)
              }
              frame "Reset" {
                n144 = for {
                  shift-right: [w361] -> w356
                  shift-left: w357 -> [w362]
                  tunnel: string[] ["Software reset", "Hardware reset", ""] -> [w360] mode=indexing
                  n145 = Enqueue Element(queue=w362, element=w360) -> (queue out=w361:refnum<queue>)  [unwired: 2 in, 2 out]
                }
                n146 = Wait (ms)(milliseconds to wait=u32 250) -> ()  [unwired: 1 out]
              }
              frame "Processing" {
              }
              frame "Shutdown" {
                # ">>State Logic >>"
                n147 = for {
                  shift-right: [w370] -> w365
                  shift-left: w366 -> [w371]
                  tunnel: string[] ["Software reset", "Hardware reset", "Cam Exit", "Exit"] -> [w369] mode=indexing
                  n148 = Enqueue Element(queue=w371, element=w369) -> (queue out=w370:refnum<queue>)  [unwired: 2 in, 2 out]
                }
              }
              frame "None" {
              }
              frame "Task 4e" {
              }
              frame "Task 4f" {
              }
              frame "Task 4g" {
              }
              frame "Task 4h" {
              }
              frame "Wall follow mode" {
                n149 = case shown="True" w382 {
                  tunnel: [string[] ["IR Sensor Read", "Calculate", "Forward", "Motor Control"] string[] ["Hardware reset", "Software reset", "Motor Control"]] -> w383
                  frame False {
                  }
                  frame True {
                  }
                }
                n150 = for {
                  shift-right: [w392] -> w385
                  shift-left: w384 -> [w393]
                  tunnel: w383 -> [w391] mode=indexing
                  n151 = Enqueue Element(queue=w393, element=w391) -> (queue out=w392:refnum<queue>)  [unwired: 2 in, 2 out]
                }
                n152 = Select(t=TLB_MHL_States."Idle" ("Enum"), s=w382, f=TLB_MHL_States."Wall follow mode" ("Enum")) -> (s? t:f=w387:T11)
              }
              frame "Acquire image" {
                n153 = case shown="False" w394 {
                  tunnel: [_ string[] ["Hardware reset", "Software reset", "Cam Exit", ""]] -> w398
                  frame False {
                  }
                  frame True {
                  }
                }
                n154 = for {
                  shift-right: [w403] -> w396
                  shift-left: w397 -> [w404]
                  tunnel: w398 -> [w402] mode=indexing
                  n155 = Enqueue Element(queue=w404, element=w402) -> (queue out=w403:refnum<queue>)  [unwired: 2 in, 2 out]
                }
                n156 = Select(t=TLB_MHL_States."Idle" ("Enum"), s=w394, f=TLB_MHL_States."Acquire image" ("Enum")) -> (s? t:f=w395:T11)
              }
            }
          }
        }
      }
      n157 = while {
        stop <- w121 stop-if-true
        # "Motor control loop"
        n158 = call "FGV Bool.vi"("Init/Read/Write State"=States_for_Action_Engine."Read") -> ("Output node"=w121:bool)  [unwired: 2 in, 1 out]
        n159 = call "New motor Control integrated.vi"("wTargetSpeed"="wTargetSpeed", "yTargetSpeed"="yTargetSpeed", "xTargetSpeed"="Reset Encoder 0", "Reset Encoders"="xTargetSpeed") -> ("Speed"=→"Speed":T10, "Distance"=→"Distance":T9)
      }
      n160 = while {
        tunnel: [w91] -> w19
        tunnel: [w88] -> w18
        tunnel: [w87] -> w16
        tunnel: [w86] -> w17
        tunnel: [w83] -> w15
        stop <- w93 stop-if-true
        # "NavX Loop"
        n161 = call <vilib>:"NavX Open.vi"("I2C Channel"=I2C_Channel."A") -> ("NavX Info"=w84:T5)  [unwired: 9 in, 1 out]
        n162 = case shown="True" "NavX Zero Yaw" {
          tunnel: w84 -> [w95 w97]
          tunnel: [w95 w96] -> w83
          frame False {
          }
          frame True {
            n163 = call <vilib>:"Zero Yaw.vi"("NavX Info In"=w97) -> ("NavX Info Out"=w96:T5)  [unwired: 10 in]
          }
        }
        n164 = call <vilib>:"YRPHfH.vi"("NavX Info In"=w84) -> ("YRPHfH"=w81:T8, "NavX Info Out"=w87:T5)  [unwired: 3 in]
        "YRPHfH" <- w81
        n165 = call <vilib>:"Raw Values.vi"("NavX Info In"=w84) -> ("NavX Info Out"=w91:T5)  [unwired: 8 in, 1 out]
        "NavX Info Out" <- w91
        n166 = call <vilib>:"LinearAcceleration.vi"("NavX Info In"=w84) -> ("LinearAcceleration"=→"LinearAcceleration":T6, "NavX Info Out"=w88:T5)  [unwired: 9 in]
        n167 = call <vilib>:"Displacement.vi"("NavX Info In"=w84) -> ("Displacement"=→"Displacement":T7, "NavX Info Out"=w86:T5)  [unwired: 9 in]
        n168 = Unbundle By Name(w81) -> ("Yaw"=→"Yaw":dbl)
        n169 = call "FGV Bool.vi"("Init/Read/Write State"=States_for_Action_Engine."Read") -> ("Output node"=w93:bool)  [unwired: 2 in, 1 out]
        n170 = Wait Until Next ms Multiple(millisecond multiple=u32 10) -> ()  [unwired: 1 out]
      }
      n171 = while {
        stop <- w73 stop-if-true
        # "Blackhawk interfacing"
        n172 = call <vilib>:"Blackhawk i2c Open.vi"("I2C Channel"=I2C_Channel."B") -> ("I2C Ref Out"=w79:T18, "error out"=w78:errorcluster)  [unwired: 2 in]
        n173 = call <vilib>:"Blackhawk DIO Read.vi"("I2C Ref In"=w79, "PIN"=u8 0, "error in (no error)"=w78) -> ("I2C Ref Out"=w71:T18, "Value Read"=→"Value Read":bool, "error out"=w72:errorcluster)  [unwired: 3 in]
        n174 = call <vilib>:"Blackhawk Relay.vi"("error in (no error)"=w72, "On/Off"="On/Off", "Relay"=enum8{"Relay 0", "Relay 1", "Relay 2"}."Relay 0", "I2C Ref In"=w71) -> ("error out"=w67:errorcluster, "I2C Ref Out"=w68:T18)  [unwired: 6 in]
        n175 = call <vilib>:"Blackhawk Servo.vi"("error in (no error)"=w67, "Servo Select"=enum16{"Servo 5", "Servo 6"}."Servo 5", "Servo Angle"="Servo Angle", "I2C Ref In"=w68) -> ("error out"=→"Blackhawk error":errorcluster)  [unwired: 6 in, 1 out]
        n176 = call <vilib>:"Blackhawk Servo.vi"() -> ()  [unwired: 10 in, 2 out]
        n177 = call "FGV Bool.vi"("Init/Read/Write State"=States_for_Action_Engine."Read") -> ("Output node"=w73:bool)  [unwired: 2 in, 1 out]
      }
      n178 = while {
        shift-right: [w102] -> _
        shift-left: _ -> [w103]
        stop <- w108 stop-if-true
        w113 = T19 [enum."B/AI0"] items=["Not Connected", "AudioIn/Left", "AudioIn/Right", "C/AI0", "C/AI1", "A/AI0", "A/AI1", "A/AI2", "A/AI3", "A/AI4", "A/AI5", "A/AI6", "A/AI7", "B/AI0", "B/AI1", "B/AI2", "B/AI3", "B/AI4", "B/AI5", "B/AI6", "B/AI7", "AI/AI0", "AI/AI1", "AI/AI2", "AI/AI3", "A/AI0 (DIFF)", "A/AI1 (DIFF)", "A/AI2 (DIFF)", "A/AI3 (DIFF)", "B/AI0 (DIFF)", "B/AI1 (DIFF)", "B/AI2 (DIFF)", "B/AI3 (DIFF)"] ("AI Channel")
        w114 = T19 [enum."A/AI0"] items=["Not Connected", "AudioIn/Left", "AudioIn/Right", "C/AI0", "C/AI1", "A/AI0", "A/AI1", "A/AI2", "A/AI3", "A/AI4", "A/AI5", "A/AI6", "A/AI7", "B/AI0", "B/AI1", "B/AI2", "B/AI3", "B/AI4", "B/AI5", "B/AI6", "B/AI7", "AI/AI0", "AI/AI1", "AI/AI2", "AI/AI3", "A/AI0 (DIFF)", "A/AI1 (DIFF)", "A/AI2 (DIFF)", "A/AI3 (DIFF)", "B/AI0 (DIFF)", "B/AI1 (DIFF)", "B/AI2 (DIFF)", "B/AI3 (DIFF)"] ("AI Channel")
        # "IR + Ultrasonic Sensor Loop"
        n179 = call <vilib>:"Ping.vi"("Mxp Side"=Mxp_Selection."MXP B") -> ("CM"=w101:fxp<+,64,16>)  [unwired: 8 in, 2 out]
        "CM" <- w101
        n180 = call <vilib>:"Sharp IR.vi"("AI Channel"=w114) -> ("Sharp IR Distance"=→"Right IR Sensor":dbl)  [unwired: 8 in, 2 out]
        n181 = call <vilib>:"Sharp IR.vi"("AI Channel"=w113) -> ("Sharp IR Distance"=→"Left IR Sensor":dbl)  [unwired: 8 in, 2 out]
        n182 = Greater Or Equal?(x=w101, y=fxp<+,64,16> 299.0) -> (x >= y?=w104:bool)
        n183 = call <vilib>:"Mean PtByPt.vi"("x"=w101, "sample length"=100) -> ()  [unwired: 2 in, 2 out]
        n184 = Select(t=w103, s=w104, f=w101) -> (s? t:f=w102:fxp<+,64,16>)
        "Ultrasonic sensor" <- w102
        n185 = call "FGV Bool.vi"("Init/Read/Write State"=States_for_Action_Engine."Read") -> ("Output node"=w108:bool)  [unwired: 2 in, 1 out]
        n186 = In Range and Coerce(upper limit=fxp<+,64,16> 250.0, x=w101, lower limit=fxp<+,64,16> 0.0 ("CM")) -> ()  [unwired: 2 out]
        n187 = Wait Until Next ms Multiple(millisecond multiple=u32 10) -> ()  [unwired: 1 out]
      }
      n188 = call <vilib>:"IMAQdx Open Camera.vi"("Session In"=T13 "cam1") -> ("error out"=w5:errorcluster, "Session Out"=w4:T13)  [unwired: 9 in]
      n189 = call "IMAQ Create"("Image Name"="image") -> ("New Image"=w12:T2, "error out"=w11:errorcluster)  [unwired: 4 in]
      n190 = call <vilib>:"IMAQdx Configure Grab.vi"("error in"=w5, "Session In"=w4) -> ("error out"=w2:errorcluster, "Session Out"=w3:T13)  [unwired: 8 in]
      n191 = while {
        tunnel: w12 -> [w50]
        tunnel: w11 -> [w56]
        tunnel: [w57] -> w8
        tunnel: [w50] -> w10
        tunnel: [w54] -> w9
        tunnel: [w54] -> w7
        tunnel: w3 -> [w52]
        tunnel: w2 -> [w51]
        stop <- w62 stop-if-true
        # "Webcam loop"
        n192 = call <vilib>:"IMAQdx Grab2.vi"("error in"=w51, "Image In"=w50, "Session In"=w52) -> ("error out"=w59:errorcluster, "Image Out"=w55:T2, "Session Out"=w57:T13)  [unwired: 5 in, 1 out]
        n193 = Wait (ms)(milliseconds to wait=u32 500) -> ()  [unwired: 1 out]
        n194 = call "Colour detection subVI.vi"("error in"=w59, "Enum"="Enum", "Image In"=w55) -> ("error out"=w58:errorcluster, "Image overlay"=→"Image Out":T2)
        n195 = Merge Errors(w58, w56) -> (w54:errorcluster)
        "Image Processing error" <- w54
        n196 = call "FGV Bool.vi"("Init/Read/Write State"=States_for_Action_Engine."Read") -> ("Output node"=w62:bool)  [unwired: 2 in, 1 out]
      }
      n197 = call <vilib>:"NavX Close.vi"("NavX Info In"=w15) -> ()  [unwired: 10 in, 1 out]
      n198 = call <vilib>:"NavX Close.vi"("NavX Info In"=w19) -> ()  [unwired: 10 in, 1 out]
      n199 = call <vilib>:"NavX Close.vi"("NavX Info In"=w18) -> ()  [unwired: 10 in, 1 out]
      n200 = call <vilib>:"NavX Close.vi"("NavX Info In"=w17) -> ()  [unwired: 10 in, 1 out]
      n201 = call <vilib>:"NavX Close.vi"("NavX Info In"=w16) -> ()  [unwired: 10 in, 1 out]
      n202 = call <vilib>:"IMAQdx Close Camera.vi"("error in"=w7, "Session In"=w8) -> ()  [unwired: 9 in, 1 out]
      n203 = call "Imaq Dispose"("Image"=w10, "error in (no error)"=w9) -> ()  [unwired: 4 in, 1 out]
      n204 = Merge Errors "Merge Errors"(w43, w42) -> (w22:errorcluster)
      n205 = Merge Errors(w28, w22) -> (w24:errorcluster)
      n206 = Destroy User Event(user event=w46, error in=w24) -> ()  [unwired: 1 out]
      n207 = Destroy User Event(user event=w47, error in=w24) -> ()  [unwired: 1 out]
      n208 = Unregister For Events(event registration refnum=w38, error in=w24) -> ()  [unwired: 1 out]
      n209 = Release Queue(queue=w37, error in (no error)=w24) -> ()  [unwired: 1 in, 3 out]
      n210 = Release Queue(queue=w23, error in (no error)=w24) -> ()  [unwired: 1 in, 3 out]
    }
    frame #2 {
    }
  }
